vi "5.PID-Host GUI.vi"() -> ()   [LabVIEW 2014]
doc: "This example demonstrates how to implement a STM client which receives messages from the server.\n\nThe server needs to be started before the client."
uses:
  vi.lib/Q-WaveSystems/QwaveSys Raspberry Pi for LabVIEW Home-Education/STM/TCP/STM Read Meta Data (TCP Ref).vi
  vi.lib/Q-WaveSystems/QwaveSys Raspberry Pi for LabVIEW Home-Education/STM/TCP/STM Read Message (TCP).vi
  vi.lib/Q-WaveSystems/QwaveSys Raspberry Pi for LabVIEW Home-Education/STM/TCP/STM Get Connection Reference (TCP).vi
  vi.lib/Q-WaveSystems/QwaveSys Raspberry Pi for LabVIEW Home-Education/QwaveSys Raspberry Pi Library.lvlib
panel:
  out "Output (MV)":dbl(graph)
  out "Alarm Higher Limit":bool
  out "Alarm Lower Limit":bool
  out "Max":dbl
  out "Min":dbl
  out "SP":dbl
  out "PV":dbl
  out "Monitor Chart":cluster{"initial PV":dbl, "SP:":dbl, dbl, dbl}(graph)
  out "error  out":errorcluster
  in  "Target IP Address":string="192.168.5.1"
  in  "stop":bool
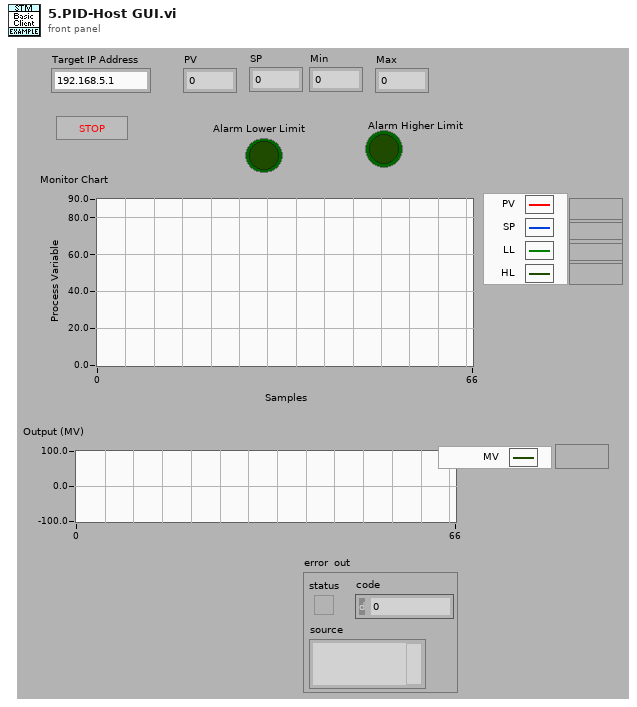
[diagram p1: front panel]
types:
  T1 = typedef "QwaveSys Raspberry Pi Library.lvlib/stm_TCP Connection Info.ctl" = cluster{"connection ID":refnum<k5>, "Meta data":T2[]}
  T2 = typedef "QwaveSys Raspberry Pi Library.lvlib/stm_MetaDataElement.ctl" = string
  T3 = cluster{"PV":dbl, "SP":dbl, "Min":dbl, "Max":dbl}
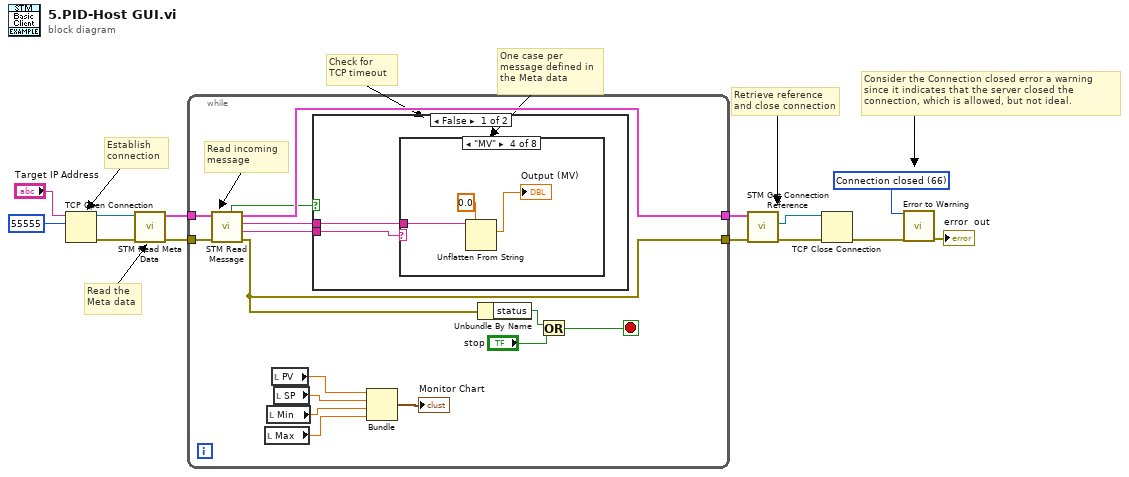
[diagram p0: block diagram]
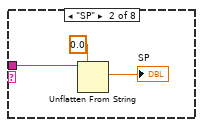
[diagram p3: hidden frame]
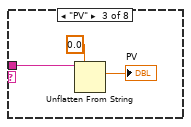
[diagram p4: hidden frame]
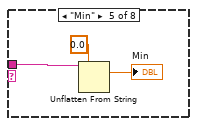
[diagram p5: hidden frame]
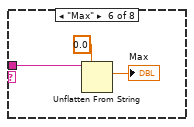
[diagram p6: hidden frame]
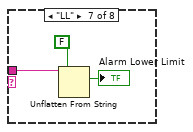
[diagram p7: hidden frame]
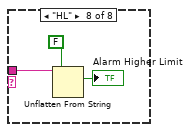
[diagram p8: hidden frame]
diagram:
  w7 = 66 items=["No Error", "Argument Error", "Memory Full", "Out of Zone", "End of File", "File Already Open", "Generic File IO Error", "File Not Found", "File Permission Error", "Disk Full", "Duplicate Path", "Too Many Files Open", "Not Enabled", "Resource File Not Found", "Cannot Add Resource", "Resource Not Found", "Image Not Found", "Image Memory Error", "Pen Does Not Exist", "Config Bad Type", "Config Token Not Found", "Config Parse Error", "Config Memory Error", "Bad External Code Format", "Bad External Code Offset", "External Code Not Present", "Null Window", "Destroy Window Mixup", "Null Menu", "Print Aborted", "Bad Print Record", "Print Driver Error", "Windows Error During Print", "Memory Error During Print", "Print Dialog Error", "Generic Print Error", "Invalid Device Refnum", "Device Not Found", "Device Parameter Error", "Device Unit Error", "Can't Open Device", "Device Call Aborted", "Generic Error", "Cancelled By User", "Object ID Too Low", "Object ID Too High", "Object Not In Heap", "Unknown Heap", "Bad DefProc ID", "DefProc Not In Table", "Message Out Of Range", "Null Method", "Unknown Message", "Manager Call Not Supported", "Bad address", "Connection In progress", "Connection timed out", "Connection is already in progress", "Network attribute not supported", "Network error", "Address in use", "System out of memory", "Connection aborted", "Connection refused", "Connection is not connected", "Connection is already connected", "Connection closed", "Initialize error (interapplication manager)", "Bad occurrence", "Wait on unbound occurrence handler", "Occurrence queue overflow", "Bad path", "Semaphore not signaled", "Unrecognized type (interapplication manager)"] ("1st Error to Convert")
  # "Consider the Connection closed error a warning since it indicates that the server closed the connection, which is allowed, but not ideal."
  # "Retrieve reference and close connection"
  # "Check for\nTCP timeout"
  # "One case per\nmessage defined in\nthe Meta data"
  # "Read the \nMeta data"
  # "Establish\nconnection"
  n1 = TCP Open Connection(address="Target IP Address", remote port or service name=u16 55555 ("remote port")) -> (connection ID=w13:refnum<k5>, error out=w11:errorcluster)  [unwired: 1 in, 2 out]
  n2 = call-poly "STM Read Meta Data.vi"("error in"=w11, "connection ID"=w13) -> ("error out"=w10:errorcluster, "Connection Info Out"=w12:T1)  [unwired: 1 in, 7 out]
  n3 = while {
    tunnel: w12 -> [w28]
    tunnel: w10 -> [w27]
    tunnel: [w26] -> w4
    tunnel: [w23] -> w3
    stop <- w20 stop-if-true
    # "Read incoming\nmessage"
    n4 = call-poly "STM Read Message.vi"("error in"=w27, "Connection Info"=w28) -> ("error out"=w23:errorcluster, "Name"=w25:T2, "data string"=w24:string, "Connection Info Out"=w26:T1, "Timed Out?"=w19:bool)  [unwired: 1 in, 4 out]
    n5 = local read "Max"() -> (w14:dbl)
    n6 = local read "Min"() -> (w15:dbl)
    n7 = local read "PV"() -> (w17:dbl)
    n8 = local read "SP"() -> (w16:dbl)
    n9 = case shown="False" w19 {
      tunnel: w25 -> [w29 _]
      tunnel: w24 -> [w30 _]
      frame False {
        n10 = case shown="\"MV\"" w29 {
          tunnel: w30 -> [_ w31 w34 w38 w40 w43 w48 w51]
          frame Default {
          }
          frame "SP" {
            n11 = Unflatten From String(type=0.0, binary string=w31) -> (value=→"SP":dbl)  [unwired: 1 in, 4 out]
          }
          frame "PV" {
            n12 = Unflatten From String(type=0.0, binary string=w34) -> (value=→"PV":dbl)  [unwired: 1 in, 4 out]
          }
          frame "MV" {
            n13 = Unflatten From String(type=0.0, binary string=w38) -> (value=→"Output (MV)":dbl)  [unwired: 1 in, 4 out]
          }
          frame "Min" {
            n14 = Unflatten From String(type=0.0, binary string=w40) -> (value=→"Min":dbl)  [unwired: 1 in, 4 out]
          }
          frame "Max" {
            n15 = Unflatten From String(type=0.0, binary string=w43) -> (value=→"Max":dbl)  [unwired: 1 in, 4 out]
          }
          frame "LL" {
            n16 = Unflatten From String(type=FALSE, binary string=w48) -> (value=→"Alarm Lower Limit":bool)  [unwired: 1 in, 4 out]
          }
          frame "HL" {
            n17 = Unflatten From String(type=FALSE, binary string=w51) -> (value=→"Alarm Higher Limit":bool)  [unwired: 1 in, 4 out]
          }
        }
      }
      frame True {
      }
    }
    n18 = Bundle("PV"=w17, "SP"=w16, "Min"=w15, "Max"=w14) -> (→"Monitor Chart":T3)  [unwired: 1 in]
    n19 = Unbundle By Name(w23) -> ("status"=w22:bool)
    n20 = Or(x=w22, y="stop") -> (x .or. y?=w20:bool)
  }
  n21 = call-poly "STM Get Connection Reference.vi"("error in"=w3, "Connection Info"=w4) -> ("error out"=w1:errorcluster, "connection ID out"=w2:refnum<k5>)  [unwired: 8 out]
  n22 = TCP Close Connection(connection ID=w2, error in (no error)=w1) -> (error out=w6:errorcluster)  [unwired: 2 out]
  n23 = call <vilib>:"Error to Warning.vi"("1st Error to Convert"=w7, "error in"=w6) -> ("warning out"=→"error  out":errorcluster)  [unwired: 3 in, 10 out]
